vi "Untitled 1.vi"() -> ()   [LabVIEW 2020]
panel:
  in  "Tab Control":enum32{"Page 2"}(tab)
  in  "Initial Value":dbl
  in  "value":bool
  in  "Final Value":dbl
  out "Current Result":dbl
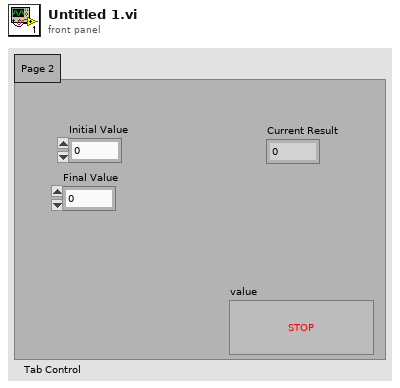
[diagram p1: front panel]
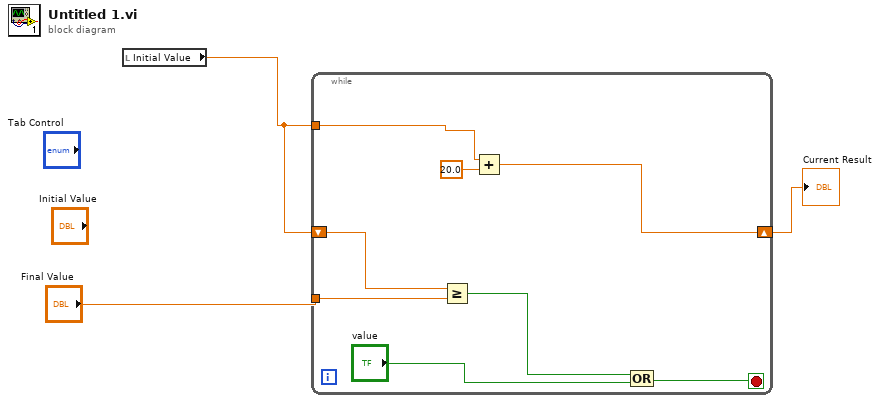
[diagram p0: block diagram]
diagram:
  n1 = local read "Initial Value"() -> (w1:dbl)
  n2 = while {
    shift-right: [w5] -> w2
    shift-left: w1 -> [w8]
    tunnel: "Final Value" -> [w6]
    tunnel: w1 -> [w4]
    stop <- w11 stop-if-true
    n3 = Greater Or Equal?(x=w8, y=w6) -> (x >= y?=w10:bool)
    n4 = Add(x=w4, y=20.0) -> (x+y=w5:dbl)
    n5 = Compound Arithmetic op=OR(w10, "value") -> (w11:bool)
  }
  "Current Result" <- w2
